vi "LF Write File (I32)__ogtk.vi"(5 "data":i32[](array[numeric]), 7 "error in (no error)":errorcluster, 8 "offset in (0)":dbl, 9 "pos mode (current)":enum16{"start", "end", "current"}(ring)=enum."current", 10 "refnum":refnum<file>) -> (0 "error out":errorcluster, 1 "offset out":dbl, 3 "refnum out":refnum<file>)   [LabVIEW 2012]
doc: "Writes an array of 32 bit integers using a double precision number as offset to work for files larger than 2GB."
uses:
  kernel32.dll
panel:
  # "max offset is limited to about\n2^51 (1 000 000 000 000 000)  bytes\nto maintain full resolution of 1 bytes"
  # "LF Write File (I32).vi\n\nPlease visit http://www.OpenG.org to learn about the\nOpen Source LabVIEW software movement.\n\nNOTICE -- YOU MUST LEAVE THIS NOTICE IN PLACE.  PER THE TERMS OF THE LICENSE BELOW, YOU MAY SUBLICENSE THIS SOFTWARE \nIN ANY WAY THAT DOES NOT CONFLICT WITH THIS LICENSE.\n\n### BSD License (http://www.opensource.org/licenses/bsd-license.php) Begin ###\n\nCopyright (c) 2003, Rolf Kalbermatter <rolf.kalbermatter@citeng.com>\n\nAll rights reserved.\n\nRedistribution and use in source and binary forms, with or without modification, are permitted provided that the following conditions are met:\n\n    * Redistributions of source code must retain the above copyright notice, this list of conditions and the following disclaimer.\n    * Redistributions in binary form must reproduce the above copyright notice, this list of conditions and the following disclaimer in the \n       documentation and/or other materials provided with the distribution.\n    * Neither the name of SciWare, James Kring, Inc., nor the names of its contributors may be used to endorse or promote products derived \n       from this software without specific prior written permission.\n\nTHIS SOFTWARE IS PROVIDED BY THE COPYRIGHT HOLDERS AND CONTRIBUTORS \"AS IS\" AND ANY EXPRESS OR IMPLIED WARRANTIES, \nINCLUDING, BUT NOT LIMITED TO, THE IMPLIED WARRANTIES OF MERCHANTABILITY AND FITNESS FOR A PARTICULAR PURPOSE ARE \nDISCLAIMED. IN NO EVENT SHALL THE COPYRIGHT OWNER OR CONTRIBUTORS BE LIABLE FOR ANY DIRECT, INDIRECT, INCIDENTAL,\n SPECIAL, EXEMPLARY, OR CONSEQUENTIAL DAMAGES (INCLUDING, BUT NOT LIMITED TO, PROCUREMENT OF SUBSTITUTE GOODS OR \nSERVICES; LOSS OF USE, DATA, OR PROFITS; OR BUSINESS INTERRUPTION) HOWEVER CAUSED AND ON ANY THEORY OF LIABILITY, \nWHETHER IN CONTRACT, STRICT LIABILITY, OR TORT (INCLUDING NEGLIGENCE OR OTHERWISE) ARISING IN ANY WAY OUT OF THE USE \nOF THIS SOFTWARE, EVEN IF ADVISED OF THE POSSIBILITY OF SUCH DAMAGE.\n\n### BSD License End ###"
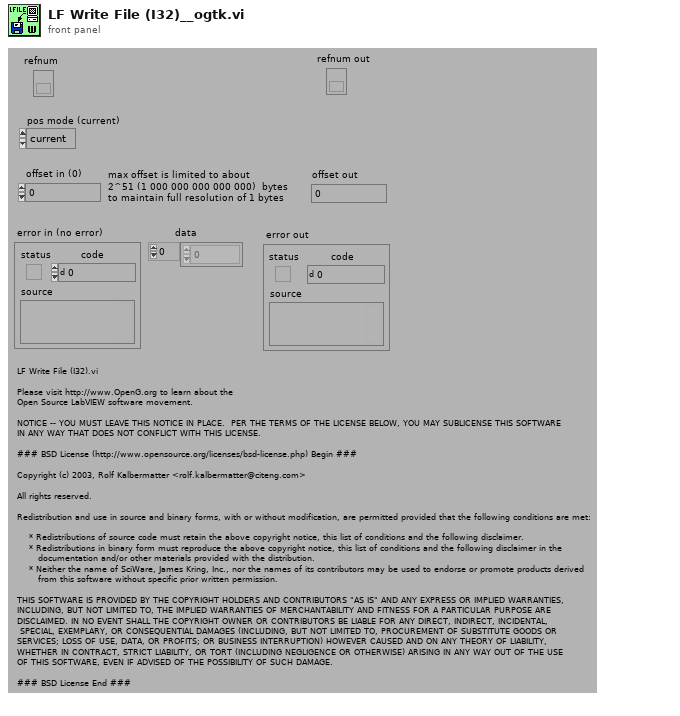
[diagram p1: front panel]
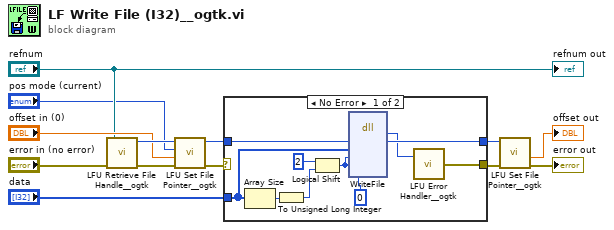
[diagram p0: block diagram]
diagram:
  n1 = call <userlib>:"LFU Retrieve File Handle__ogtk.vi"("error in (no error)"="error in (no error)", "file refnum"="refnum") -> ("error out"=w11:errorcluster, "handle out"=w12:u32)  [unwired: 4 in]
  n2 = call <userlib>:"LFU Set File Pointer__ogtk.vi"("error in (no error)"=w11, "offset in (0)"="offset in (0)", "pos mode (current)"="pos mode (current)", "handle"=w12) -> ("error out"=w3:errorcluster, "handle out"=w6:u32)  [unwired: 1 in, 1 out]
  n3 = case shown="No Error" w3 {
    selector: w3 -> [_ w25]
    tunnel: w6 -> [w22 w24]
    tunnel: "data" -> [w21 _]
    tunnel: [w20 w24] -> w2
    tunnel: [w18 w25] -> w1
    frame No Error {
      n4 = Array Size(array=w21) -> (size(s)=w19:i32)
      n5 = To Unsigned Long Integer(number=w19) -> (unsigned 32bit integer=w16:u32)
      n6 = Logical Shift(y=2, x=w16) -> (x << y=w14:u32)
      n7 = dll-call lib="kernel32.dll" fn="WriteFile"("handle"=w22, "buffer"=w21, "bytesToRead"=w14, "bytesRead"=w14, "overlapped"=u32 0) -> (w17:u32, "handle"=w20:u32)  [unwired: 7 in, 2 out]
      n8 = call <userlib>:"LFU Error Handler__ogtk.vi"("retval"=w17) -> ("error out"=w18:errorcluster)  [unwired: 1 in]
    }
    frame Error {
    }
  }
  n9 = call <userlib>:"LFU Set File Pointer__ogtk.vi"("error in (no error)"=w1, "handle"=w2) -> ("error out"=→"error out":errorcluster, "offset out"=→"offset out":dbl)  [unwired: 3 in, 1 out]
  "refnum out" <- "refnum"
